vi "SME Reader.vi"() -> ()   [LabVIEW 2020]
uses:
  Accumulator/Accumulator.lvclass
  Data/Data.lvclass
panel:
  out "End?":bool
  out "Inside?":bool
  out "Temp_Graph":dbl(graph)
  out "Current_String":string
  out "Char":string
  in  "stop":bool
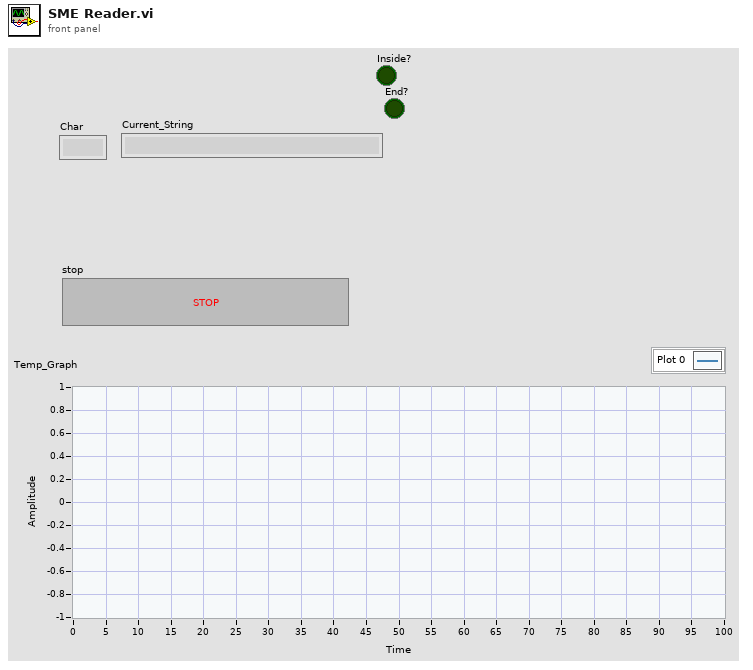
[diagram p1: front panel]
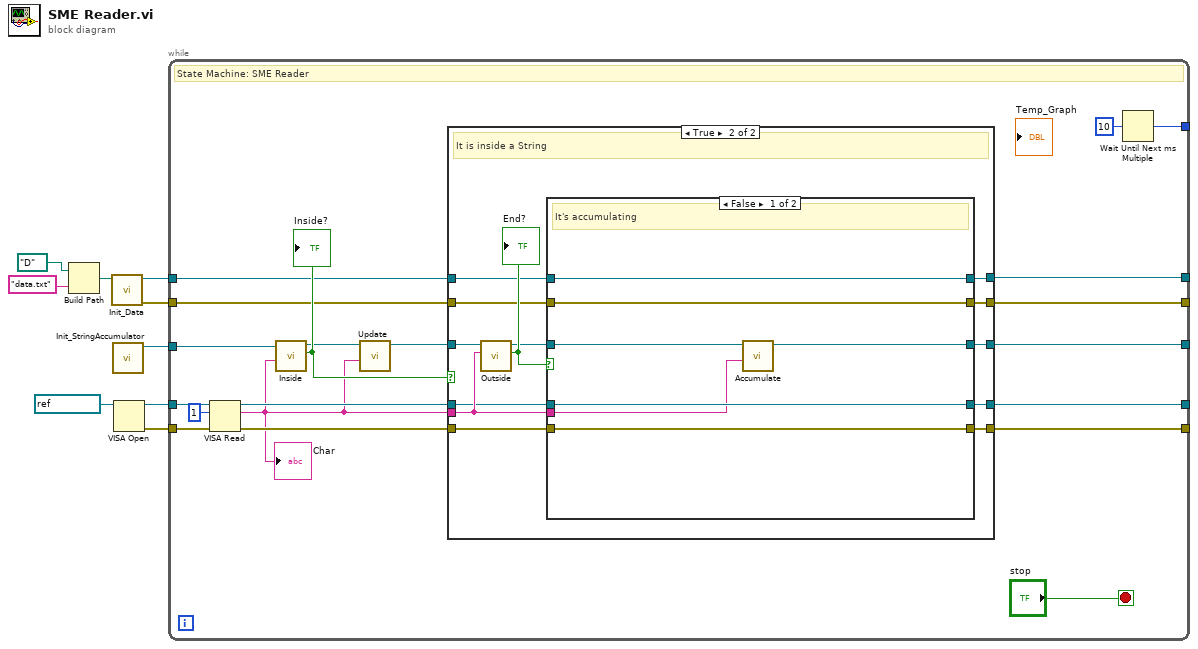
[diagram p0: block diagram]
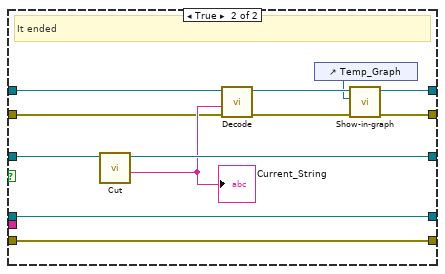
[diagram p3: hidden frame]
diagram:
  n1 = Build Path(base path=path "D:/", name or relative path="data.txt") -> (appended path=w2:path)
  n2 = call "Init_Data.vi"("datalog path"=w2) -> ("error out"=w5:errorcluster, "Data"=w4:refnum<class "Data.lvclass">)  [unwired: 9 in]
  n3 = call "Init_StringAccumulator.vi"() -> ("Accumulator"=w9:refnum<class "Accumulator.lvclass">)  [unwired: 11 in]
  n4 = VISA Open(VISA resource name=refnum<visa-resource-name> "CNCB0") -> (VISA resource name=w8:refnum<visa-resource-name>, error out=w7:errorcluster)  [unwired: 4 in]
  n5 = while {
    tunnel: w9 -> [w29]
    tunnel: w8 -> [w27]
    tunnel: w7 -> [w26]
    tunnel: [w25] -> _
    tunnel: [w22] -> _
    tunnel: w5 -> [w20]
    tunnel: w4 -> [w19]
    tunnel: [w18] -> _
    tunnel: [w16] -> _
    tunnel: [w14] -> _
    tunnel: [w13] -> _
    stop <- "stop" stop-if-true
    # "State Machine: SME Reader"
    n6 = VISA Read(VISA resource name=w27, byte count=u32 1, error in (no error)=w26) -> (VISA resource name out=w17:refnum<visa-resource-name>, read buffer=w11:string, error out=w15:errorcluster)  [unwired: 1 out]
    "Char" <- w11
    n7 = call "Inside.vi"("Current_char"=w11, "Accumulator"=w29) -> ("Inside?"=w23:bool, "Accumulator'"=w12:refnum<class "Accumulator.lvclass">)  [unwired: 8 in]
    "Inside?" <- w23
    n8 = call "Update.vi"("Char"=w11, "Accumulator"=w12) -> ("Accumulator'"=w10:refnum<class "Accumulator.lvclass">)  [unwired: 9 in]
    n9 = case shown="True" w23 {
      tunnel: w10 -> [w30 w47]
      tunnel: w11 -> [_ w43]
      tunnel: [w30 w44] -> w22
      tunnel: w20 -> [w33 w42]
      tunnel: w19 -> [w34 w41]
      tunnel: [w32 w40] -> w18
      tunnel: w17 -> [w32 w39]
      tunnel: [w34 w38] -> w16
      tunnel: w15 -> [w31 w37]
      tunnel: [w31 w36] -> w14
      tunnel: [w33 w35] -> w13
      frame False {
        # "It has not yet started"
      }
      frame True {
        # "It is inside a String"
        n10 = call "Outside.vi"("Current_char"=w43, "Accumulator"=w47) -> ("End?"=w46:bool, "Accumulator'"=w45:refnum<class "Accumulator.lvclass">)  [unwired: 8 in]
        "End?" <- w46
        n11 = case shown="False" w46 {
          tunnel: w45 -> [w50 w66]
          tunnel: [w49 w65] -> w44
          tunnel: w43 -> [w48 _]
          tunnel: w42 -> [w51 w63]
          tunnel: w41 -> [w54 w62]
          tunnel: [w53 w61] -> w40
          tunnel: w39 -> [w53 w61]
          tunnel: [w54 w56] -> w38
          tunnel: w37 -> [w52 w60]
          tunnel: [w52 w60] -> w36
          tunnel: [w51 w57] -> w35
          frame False {
            # "It's accumulating"
            n12 = call "Accumulate.vi"("Char"=w48, "Accumulator"=w50) -> ("Accumulator'"=w49:refnum<class "Accumulator.lvclass">)  [unwired: 9 in]
          }
          frame True {
            # "It ended"
            n13 = call "Cut.vi"("Accumulator"=w66) -> ("Current_String"=w64:string, "Accumulator'"=w65:refnum<class "Accumulator.lvclass">)  [unwired: 9 in]
            "Current_String" <- w64
            n14 = call "Decode.vi"("error in"=w63, "input string"=w64, "previous_Data"=w62) -> ("error out"=w58:errorcluster, "Data"=w59:refnum<class "Data.lvclass">)  [unwired: 7 in]
            n15 = control-ref of="Temp_Graph"() -> (w55:refnum<vi>)
            n16 = call "Show-in-graph.vi"("error in"=w58, "ref_Graph"=w55, "Data"=w59) -> ("error out"=w57:errorcluster, "Data'"=w56:refnum<class "Data.lvclass">)  [unwired: 7 in]
          }
        }
      }
    }
    n17 = Wait Until Next ms Multiple(millisecond multiple=u32 10) -> (millisecond timer value=w25:u32)
  }
